vi "Lab Panel V5.24.2.vi"() -> ()   [LabVIEW 2013] (continued)
                            n1486 = TDMS Write(0:w2783, 5:"TEST PASS", 7:w2787, 9:w2786) -> (15:w2789:errorcluster)  [unwired: 2 in, 3 out]
                            n1487 = local write "data file error"(w2789) -> ()
                          }
                          frame #1 {
                            n1488 = Bundle(cluster=w2790, "STATUS"="T-RISE PASS") -> (w2792:T4)  [unwired: 2 in]
                            n1489 = local write "RESULT LAB05-1"(TRUE) -> ()
                            n1490 = local write "DISP LAB05-1"(w2792) -> ()
                          }
                        }
                      }
                      frame False {
                      }
                    }
                  }
                }
              }
              frame #9 {
                # "LAB05-2"
                n1491 = Equal?(x=w2795, y=2) -> (x = y?=w2798:bool)
                n1492 = local read "DISP LAB05-2"() -> (w2800:T4)
                n1493 = Unbundle(w2800) -> ("STATUS"=w2801:string)  [unwired: 2 out]
                n1494 = Equal?(x=w2801, y="RUN") -> (x = y?=w2797:bool)
                n1495 = And(x=w2797, y=w2798) -> (x .and. y?=w2796:bool)
                n1496 = case shown="True" w2796 {
                  tunnel: w2800 -> [_ w2804]
                  tunnel: w2794 -> [_ w2807]
                  frame False {
                  }
                  frame True {
                    n1497 = local read "SET LAB05-2"() -> (w2806:T5)
                    n1498 = local read "TDMS LAB05-2"() -> (w2803:refnum<k34>)
                    n1499 = Unbundle(w2804) -> ("CYCLE"=w2808:dbl)  [unwired: 2 out]
                    n1500 = Unbundle(w2806) -> ("T-RISE mins"=w2805:dbl)  [unwired: 4 out]
                    n1501 = Greater Or Equal?(x=w2808, y=w2807) -> (x >= y?=w2809:bool)
                    n1502 = case shown="True" w2809 {
                      tunnel: w2805 -> [w2812 _]
                      tunnel: w2804 -> [w2811 _]
                      tunnel: w2803 -> [w2810 _]
                      frame True {
                        n1503 = stacked-sequence {
                          tunnel: w2812 -> [w2815 _]
                          tunnel: w2811 -> [_ w2820]
                          tunnel: w2810 -> [w2813 _]
                          frame #0 {
                            n1504 = Build Array("T-RISE") -> (w2817:string[])
                            n1505 = Build Array(w2815) -> (w2816:dbl[])
                            n1506 = TDMS Write(0:w2813, 5:"TEST PASS", 7:w2817, 9:w2816) -> (15:w2819:errorcluster)  [unwired: 2 in, 3 out]
                            n1507 = local write "data file error"(w2819) -> ()
                          }
                          frame #1 {
                            n1508 = Bundle(cluster=w2820, "STATUS"="T-RISE PASS") -> (w2822:T4)  [unwired: 2 in]
                            n1509 = local write "RESULT LAB05-2"(TRUE) -> ()
                            n1510 = local write "DISP LAB05-2"(w2822) -> ()
                          }
                        }
                      }
                      frame False {
                      }
                    }
                  }
                }
              }
            }
          }
          frame #6 {
            # "end test & close test files"
            n1511 = local read "MAIL SETTINGS"() -> (w2828:T7)
            n1512 = Unbundle(w2828) -> ("OUT SERVER ADDRESS"=w2827:string, "FROM ACCOUNT"=w2826:string)  [unwired: 5 out]
            n1513 = stacked-sequence {
              tunnel: w2838 -> [_ _ _ _ _ _ _ _ _ _]
              tunnel: w2839 -> [_ _ _ _ _ _ _ _ _ _]
              tunnel: w2837 -> [_ _ _ _ _ _ _ _ _ _]
              tunnel: w2836 -> [_ _ _ _ _ _ _ _ _ _]
              tunnel: w2835 -> [_ _ _ _ _ _ _ _ _ _]
              tunnel: w2834 -> [_ _ _ _ _ _ _ _ _ _]
              tunnel: w2833 -> [_ _ _ _ _ _ _ _ _ _]
              tunnel: w2832 -> [_ _ _ _ _ _ _ _ _ _]
              tunnel: w2831 -> [_ _ _ _ _ _ _ _ _ _]
              tunnel: w2830 -> [_ _ _ _ _ _ _ _ _ _]
              tunnel: w2827 -> [w2843 w2895 w2943 w2990 w3037 w3084 w3131 w3178 w3225 w3272]
              tunnel: w2826 -> [w2842 w2894 w2942 w2989 w3036 w3083 w3130 w3177 w3224 w3271]
              tunnel: "Mail Test File To:" -> [w2841 w2893 w2941 w2988 w3035 w3082 w3129 w3176 w3223 w3270]
              tunnel: "Mail Test Fail" -> [w2840 w2892 w2940 w2987 w3034 w3081 w3128 w3175 w3222 w3269]
              frame #0 {
                # "LAB01-1"
                n1514 = local read "DISP LAB01-1"() -> (w2847:T4)
                n1515 = local read "run lab01-1"() -> (w2844:bool)
                n1516 = local read "TDMS LAB01-1"() -> (w2845:refnum<k34>)
                n1517 = Unbundle(w2847) -> ("CYCLE"=w2848:dbl, "STATUS"=w2846:string)  [unwired: 1 out]
                n1518 = case shown="True" w2844 {
                  tunnel: w2848 -> [_ w2854]
                  tunnel: w2847 -> [_ w2856]
                  tunnel: w2846 -> [_ w2853]
                  tunnel: w2845 -> [_ w2855]
                  tunnel: w2843 -> [_ w2852]
                  tunnel: w2842 -> [_ w2851]
                  tunnel: w2841 -> [_ w2850]
                  tunnel: w2840 -> [_ w2849]
                  frame False {
                  }
                  frame True {
                    n1519 = Not Equal?(x=w2853, y="RUN") -> (x != y?=w2857:bool)
                    n1520 = Greater?(x=w2854, y=2.0) -> (0:w2859:bool)
                    n1521 = And(x=w2859, y=w2857) -> (x .and. y?=w2858:bool)
                    n1522 = case shown="True" w2858 {
                      tunnel: w2856 -> [_ w2869]
                      tunnel: w2855 -> [_ w2868]
                      tunnel: w2854 -> [_ w2867]
                      tunnel: w2853 -> [_ w2866]
                      tunnel: w2852 -> [_ w2865]
                      tunnel: w2851 -> [_ w2864]
                      tunnel: w2850 -> [_ w2863]
                      tunnel: w2849 -> [_ w2862]
                      frame False {
                      }
                      frame True {
                        n1523 = stacked-sequence {
                          tunnel: w2869 -> [w2873 _ _]
                          tunnel: w2868 -> [_ w2875 _]
                          tunnel: w2867 -> [_ _ _]
                          tunnel: w2866 -> [_ _ w2881]
                          tunnel: w2865 -> [_ _ w2880]
                          tunnel: w2864 -> [_ _ w2879]
                          tunnel: w2863 -> [_ _ w2878]
                          tunnel: w2862 -> [_ _ w2877]
                          frame #0 {
                            w2870 = FALSE
                            n1524 = local write "mail control"("END") -> ()
                            n1525 = Bundle(cluster=w2873) -> (w2872:T4)  [unwired: 3 in]
                            n1526 = local write "DISP LAB01-1"(w2872) -> ()
                            n1527 = local write "O/I  LAB01-1"(w2870) -> ()
                            n1528 = local write "run lab01-1"(w2870) -> ()
                            n1529 = local write "RUN LAB01-1"(w2870) -> ()
                          }
                          frame #1 {
                            n1530 = TDMS Close(11:w2875) -> (0:w2874:errorcluster)  [unwired: 1 in, 1 out]
                            n1531 = local write "data file error"(w2874) -> ()
                          }
                          frame #2 {
                            n1532 = stacked-sequence {
                              tunnel: "LAB01-1" -> [w2883 w2885 _]
                              tunnel: w2881 -> [_ w2891 _]
                              tunnel: w2880 -> [_ w2890 _]
                              tunnel: w2879 -> [_ w2889 _]
                              tunnel: w2878 -> [_ w2888 _]
                              tunnel: w2877 -> [_ w2887 _]
                              frame #0 {
                                n1533 = call "sub vi - defrag tdms v1.vi"("panel id"=w2883) -> ("error out"=w2882:errorcluster)  [unwired: 10 in]
                                n1534 = local write "data file error"(w2882) -> ()
                              }
                              frame #1 {
                                n1535 = Bundle("STATUS"=w2891, "OUT SERVER ADDRESS"=w2890, "FROM ACCOUNT"=w2889, "Mail Test File To:"=w2888, "Mail Test Fail"=w2887) -> (w2884:T26)  [unwired: 1 in]
                                n1536 = call "Save data file (pass-fail) v5.vi"("Input Cluster"=w2884, "panel id"=w2885) -> ("network file save error"=w2886:errorcluster)  [unwired: 8 in, 1 out]
                                n1537 = local write "data file error"(w2886) -> ()
                              }
                              frame #2 {
                              }
                            }
                          }
                        }
                      }
                    }
                  }
                }
              }
              frame #1 {
                # "LAB01-2"
                n1538 = local read "run lab01-2"() -> (w2896:bool)
                n1539 = case shown="True" w2896 {
                  tunnel: w2895 -> [_ w2900]
                  tunnel: w2894 -> [_ w2899]
                  tunnel: w2893 -> [_ w2898]
                  tunnel: w2892 -> [_ w2897]
                  frame False {
                  }
                  frame True {
                    n1540 = local read "DISP LAB01-2"() -> (w2908:T4)
                    n1541 = local read "TDMS LAB01-2"() -> (w2907:refnum<k34>)
                    n1542 = Unbundle(w2908) -> ("CYCLE"=w2902:dbl, "STATUS"=w2901:string)  [unwired: 1 out]
                    n1543 = Not Equal?(x=w2901, y="RUN") -> (x != y?=w2904:bool)
                    n1544 = Greater?(x=w2902, y=2.0) -> (0:w2905:bool)
                    n1545 = And(x=w2905, y=w2904) -> (x .and. y?=w2903:bool)
                    n1546 = case shown="True" w2903 {
                      tunnel: w2908 -> [_ w2917]
                      tunnel: w2907 -> [_ w2916]
                      tunnel: w2902 -> [_ w2915]
                      tunnel: w2901 -> [_ w2914]
                      tunnel: w2900 -> [_ w2913]
                      tunnel: w2899 -> [_ w2912]
                      tunnel: w2898 -> [_ w2911]
                      tunnel: w2897 -> [_ w2910]
                      frame False {
                      }
                      frame True {
                        n1547 = stacked-sequence {
                          tunnel: w2917 -> [w2920 _ _]
                          tunnel: w2916 -> [_ w2922 _]
                          tunnel: w2915 -> [_ _ _]
                          tunnel: w2914 -> [_ _ w2928]
                          tunnel: w2913 -> [_ _ w2927]
                          tunnel: w2912 -> [_ _ w2926]
                          tunnel: w2911 -> [_ _ w2925]
                          tunnel: w2910 -> [_ _ w2924]
                          frame #0 {
                            w2918 = FALSE
                            n1548 = local write "mail control"("END") -> ()
                            n1549 = Bundle(cluster=w2920) -> (w2921:T4)  [unwired: 3 in]
                            n1550 = local write "RUN LAB01-2"(w2918) -> ()
                            n1551 = local write "run lab01-2"(w2918) -> ()
                            n1552 = local write "O/I  LAB01-2"(w2918) -> ()
                            n1553 = local write "DISP LAB01-2"(w2921) -> ()
                          }
                          frame #1 {
                            n1554 = TDMS Close(11:w2922) -> (0:w2923:errorcluster)  [unwired: 1 in, 1 out]
                            n1555 = local write "data file error"(w2923) -> ()
                          }
                          frame #2 {
                            n1556 = stacked-sequence {
                              tunnel: "LAB01-2" -> [w2931 w2932]
                              tunnel: w2928 -> [_ w2937]
                              tunnel: w2927 -> [_ w2936]
                              tunnel: w2926 -> [_ w2935]
                              tunnel: w2925 -> [_ w2934]
                              tunnel: w2924 -> [_ w2933]
                              frame #0 {
                                n1557 = call "sub vi - defrag tdms v1.vi"("panel id"=w2931) -> ("error out"=w2930:errorcluster)  [unwired: 10 in]
                                n1558 = local write "data file error"(w2930) -> ()
                              }
                              frame #1 {
                                n1559 = Bundle("STATUS"=w2937, "OUT SERVER ADDRESS"=w2936, "FROM ACCOUNT"=w2935, "Mail Test File To:"=w2934, "Mail Test Fail"=w2933) -> (w2939:T26)  [unwired: 1 in]
                                n1560 = call "Save data file (pass-fail) v5.vi"("Input Cluster"=w2939, "panel id"=w2932) -> ("network file save error"=w2938:errorcluster)  [unwired: 8 in, 1 out]
                                n1561 = local write "data file error"(w2938) -> ()
                              }
                            }
                          }
                        }
                      }
                    }
                  }
                }
              }
              frame #2 {
                # "LAB02-1"
                n1562 = local read "run lab02-1"() -> (w2944:bool)
                n1563 = case shown="True" w2944 {
                  tunnel: w2943 -> [_ w2948]
                  tunnel: w2942 -> [_ w2947]
                  tunnel: w2941 -> [_ w2946]
                  tunnel: w2940 -> [_ w2945]
                  frame False {
                  }
                  frame True {
                    n1564 = local read "DISP LAB02-1"() -> (w2956:T4)
                    n1565 = Unbundle(w2956) -> ("CYCLE"=w2952:dbl, "STATUS"=w2949:string)  [unwired: 1 out]
                    n1566 = local read "TDMS LAB02-1"() -> (w2955:refnum<k34>)
                    n1567 = Not Equal?(x=w2949, y="RUN") -> (x != y?=w2951:bool)
                    n1568 = Greater?(x=w2952, y=2.0) -> (0:w2953:bool)
                    n1569 = And(x=w2953, y=w2951) -> (x .and. y?=w2950:bool)
                    n1570 = case shown="True" w2950 {
                      tunnel: w2956 -> [_ w2964]
                      tunnel: w2955 -> [_ w2963]
                      tunnel: w2949 -> [_ w2962]
                      tunnel: w2948 -> [_ w2961]
                      tunnel: w2947 -> [_ w2960]
                      tunnel: w2946 -> [_ w2959]
                      tunnel: w2945 -> [_ w2958]
                      frame False {
                      }
                      frame True {
                        n1571 = stacked-sequence {
                          tunnel: w2964 -> [w2967 _ _]
                          tunnel: w2963 -> [_ w2969 _]
                          tunnel: w2962 -> [_ _ w2975]
                          tunnel: w2961 -> [_ _ w2974]
                          tunnel: w2960 -> [_ _ w2973]
                          tunnel: w2959 -> [_ _ w2972]
                          tunnel: w2958 -> [_ _ w2971]
                          frame #0 {
                            w2965 = FALSE
                            n1572 = local write "mail control"("END") -> ()
                            n1573 = Bundle(cluster=w2967) -> (w2968:T4)  [unwired: 3 in]
                            n1574 = local write "O/I  LAB02-1"(w2965) -> ()
                            n1575 = local write "RUN LAB02-1"(w2965) -> ()
                            n1576 = local write "run lab02-1"(w2965) -> ()
                            n1577 = local write "DISP LAB02-1"(w2968) -> ()
                          }
                          frame #1 {
                            n1578 = TDMS Close(11:w2969) -> (0:w2970:errorcluster)  [unwired: 1 in, 1 out]
                            n1579 = local write "data file error"(w2970) -> ()
                          }
                          frame #2 {
                            n1580 = stacked-sequence {
                              tunnel: "LAB02-1" -> [w2978 w2985]
                              tunnel: w2975 -> [_ w2983]
                              tunnel: w2974 -> [_ w2982]
                              tunnel: w2973 -> [_ w2981]
                              tunnel: w2972 -> [_ w2980]
                              tunnel: w2971 -> [_ w2979]
                              frame #0 {
                                n1581 = call "sub vi - defrag tdms v1.vi"("panel id"=w2978) -> ("error out"=w2977:errorcluster)  [unwired: 10 in]
                                n1582 = local write "data file error"(w2977) -> ()
                              }
                              frame #1 {
                                n1583 = Bundle("STATUS"=w2983, "OUT SERVER ADDRESS"=w2982, "FROM ACCOUNT"=w2981, "Mail Test File To:"=w2980, "Mail Test Fail"=w2979) -> (w2984:T26)  [unwired: 1 in]
                                n1584 = call "Save data file (pass-fail) v5.vi"("Input Cluster"=w2984, "panel id"=w2985) -> ("network file save error"=w2986:errorcluster)  [unwired: 8 in, 1 out]
                                n1585 = local write "data file error"(w2986) -> ()
                              }
                            }
                          }
                        }
                      }
                    }
                  }
                }
              }
              frame #3 {
                # "LAB02-2"
                n1586 = local read "run lab02-2"() -> (w2991:bool)
                n1587 = case shown="True" w2991 {
                  tunnel: w2990 -> [_ w2995]
                  tunnel: w2989 -> [_ w2994]
                  tunnel: w2988 -> [_ w2993]
                  tunnel: w2987 -> [_ w2992]
                  frame False {
                  }
                  frame True {
                    n1588 = local read "DISP LAB02-2"() -> (w3003:T4)
                    n1589 = local read "TDMS LAB02-2"() -> (w3002:refnum<k34>)
                    n1590 = Unbundle(w3003) -> ("CYCLE"=w2999:dbl, "STATUS"=w2996:string)  [unwired: 1 out]
                    n1591 = Not Equal?(x=w2996, y="RUN") -> (x != y?=w2998:bool)
                    n1592 = Greater?(x=w2999, y=2.0) -> (0:w3000:bool)
                    n1593 = And(x=w3000, y=w2998) -> (x .and. y?=w2997:bool)
                    n1594 = case shown="True" w2997 {
                      tunnel: w3003 -> [_ w3011]
                      tunnel: w3002 -> [_ w3010]
                      tunnel: w2996 -> [_ w3009]
                      tunnel: w2995 -> [_ w3008]
                      tunnel: w2994 -> [_ w3007]
                      tunnel: w2993 -> [_ w3006]
                      tunnel: w2992 -> [_ w3005]
                      frame False {
                      }
                      frame True {
                        n1595 = stacked-sequence {
                          tunnel: w3011 -> [w3014 _ _]
                          tunnel: w3010 -> [_ w3016 _]
                          tunnel: w3009 -> [_ _ w3022]
                          tunnel: w3008 -> [_ _ w3021]
                          tunnel: w3007 -> [_ _ w3020]
                          tunnel: w3006 -> [_ _ w3019]
                          tunnel: w3005 -> [_ _ w3018]
                          frame #0 {
                            w3012 = FALSE
                            n1596 = local write "mail control"("END") -> ()
                            n1597 = Bundle(cluster=w3014) -> (w3015:T4)  [unwired: 3 in]
                            n1598 = local write "O/I  LAB02-2"(w3012) -> ()
                            n1599 = local write "run lab02-2"(w3012) -> ()
                            n1600 = local write "RUN LAB02-2"(w3012) -> ()
                            n1601 = local write "DISP LAB02-2"(w3015) -> ()
                          }
                          frame #1 {
                            n1602 = TDMS Close(11:w3016) -> (0:w3017:errorcluster)  [unwired: 1 in, 1 out]
                            n1603 = local write "data file error"(w3017) -> ()
                          }
                          frame #2 {
                            n1604 = stacked-sequence {
                              tunnel: "LAB02-2" -> [w3025 w3031]
                              tunnel: w3022 -> [_ w3030]
                              tunnel: w3021 -> [_ w3029]
                              tunnel: w3020 -> [_ w3028]
                              tunnel: w3019 -> [_ w3027]
                              tunnel: w3018 -> [_ w3026]
                              frame #0 {
                                n1605 = call "sub vi - defrag tdms v1.vi"("panel id"=w3025) -> ("error out"=w3024:errorcluster)  [unwired: 10 in]
                                n1606 = local write "data file error"(w3024) -> ()
                              }
                              frame #1 {
                                n1607 = Bundle("STATUS"=w3030, "OUT SERVER ADDRESS"=w3029, "FROM ACCOUNT"=w3028, "Mail Test File To:"=w3027, "Mail Test Fail"=w3026) -> (w3033:T26)  [unwired: 1 in]
                                n1608 = call "Save data file (pass-fail) v5.vi"("Input Cluster"=w3033, "panel id"=w3031) -> ("network file save error"=w3032:errorcluster)  [unwired: 8 in, 1 out]
                                n1609 = local write "data file error"(w3032) -> ()
                              }
                            }
                          }
                        }
                      }
                    }
                  }
                }
              }
              frame #4 {
                # "LAB03-1"
                n1610 = local read "run lab03-1"() -> (w3038:bool)
                n1611 = case shown="True" w3038 {
                  tunnel: w3037 -> [_ w3042]
                  tunnel: w3036 -> [_ w3041]
                  tunnel: w3035 -> [_ w3040]
                  tunnel: w3034 -> [_ w3039]
                  frame False {
                  }
                  frame True {
                    n1612 = local read "DISP LAB03-1"() -> (w3050:T4)
                    n1613 = local read "TDMS LAB03-1"() -> (w3049:refnum<k34>)
                    n1614 = Unbundle(w3050) -> ("CYCLE"=w3046:dbl, "STATUS"=w3043:string)  [unwired: 1 out]
                    n1615 = Not Equal?(x=w3043, y="RUN") -> (x != y?=w3045:bool)
                    n1616 = Greater?(x=w3046, y=2.0) -> (0:w3047:bool)
                    n1617 = And(x=w3047, y=w3045) -> (x .and. y?=w3044:bool)
                    n1618 = case shown="True" w3044 {
                      tunnel: w3050 -> [_ w3058]
                      tunnel: w3049 -> [_ w3057]
                      tunnel: w3043 -> [_ w3056]
                      tunnel: w3042 -> [_ w3055]
                      tunnel: w3041 -> [_ w3054]
                      tunnel: w3040 -> [_ w3053]
                      tunnel: w3039 -> [_ w3052]
                      frame False {
                      }
                      frame True {
                        n1619 = stacked-sequence {
                          tunnel: w3058 -> [w3061 _ _]
                          tunnel: w3057 -> [_ w3063 _]
                          tunnel: w3056 -> [_ _ w3069]
                          tunnel: w3055 -> [_ _ w3068]
                          tunnel: w3054 -> [_ _ w3067]
                          tunnel: w3053 -> [_ _ w3066]
                          tunnel: w3052 -> [_ _ w3065]
                          frame #0 {
                            w3059 = FALSE
                            n1620 = local write "mail control"("END") -> ()
                            n1621 = Bundle(cluster=w3061) -> (w3062:T4)  [unwired: 3 in]
                            n1622 = local write "O/I  LAB03-1"(w3059) -> ()
                            n1623 = local write "run lab03-1"(w3059) -> ()
                            n1624 = local write "RUN LAB03-1"(w3059) -> ()
                            n1625 = local write "DISP LAB03-1"(w3062) -> ()
                          }
                          frame #1 {
                            n1626 = TDMS Close(11:w3063) -> (0:w3064:errorcluster)  [unwired: 1 in, 1 out]
                            n1627 = local write "data file error"(w3064) -> ()
                          }
                          frame #2 {
                            n1628 = stacked-sequence {
                              tunnel: "LAB03-1" -> [w3072 w3078]
                              tunnel: w3069 -> [_ w3077]
                              tunnel: w3068 -> [_ w3076]
                              tunnel: w3067 -> [_ w3075]
                              tunnel: w3066 -> [_ w3074]
                              tunnel: w3065 -> [_ w3073]
                              frame #0 {
                                n1629 = call "sub vi - defrag tdms v1.vi"("panel id"=w3072) -> ("error out"=w3071:errorcluster)  [unwired: 10 in]
                                n1630 = local write "data file error"(w3071) -> ()
                              }
                              frame #1 {
                                n1631 = Bundle("STATUS"=w3077, "OUT SERVER ADDRESS"=w3076, "FROM ACCOUNT"=w3075, "Mail Test File To:"=w3074, "Mail Test Fail"=w3073) -> (w3080:T26)  [unwired: 1 in]
                                n1632 = call "Save data file (pass-fail) v5.vi"("Input Cluster"=w3080, "panel id"=w3078) -> ("network file save error"=w3079:errorcluster)  [unwired: 8 in, 1 out]
                                n1633 = local write "data file error"(w3079) -> ()
                              }
                            }
                          }
                        }
                      }
                    }
                  }
                }
              }
              frame #5 {
                # "LAB03-2"
                n1634 = local read "run lab03-2"() -> (w3085:bool)
                n1635 = case shown="True" w3085 {
                  tunnel: w3084 -> [_ w3089]
                  tunnel: w3083 -> [_ w3088]
                  tunnel: w3082 -> [_ w3087]
                  tunnel: w3081 -> [_ w3086]
                  frame False {
                  }
                  frame True {
                    n1636 = local read "DISP LAB03-2"() -> (w3097:T4)
                    n1637 = Unbundle(w3097) -> ("CYCLE"=w3093:dbl, "STATUS"=w3090:string)  [unwired: 1 out]
                    n1638 = local read "TDMS LAB03-2"() -> (w3096:refnum<k34>)
                    n1639 = Not Equal?(x=w3090, y="RUN") -> (x != y?=w3092:bool)
                    n1640 = Greater?(x=w3093, y=2.0) -> (0:w3094:bool)
                    n1641 = And(x=w3094, y=w3092) -> (x .and. y?=w3091:bool)
                    n1642 = case shown="True" w3091 {
                      tunnel: w3097 -> [_ w3105]
                      tunnel: w3096 -> [_ w3104]
                      tunnel: w3090 -> [_ w3103]
                      tunnel: w3089 -> [_ w3102]
                      tunnel: w3088 -> [_ w3101]
                      tunnel: w3087 -> [_ w3100]
                      tunnel: w3086 -> [_ w3099]
                      frame False {
                      }
                      frame True {
                        n1643 = stacked-sequence {
                          tunnel: w3105 -> [w3108 _ _]
                          tunnel: w3104 -> [_ w3110 _]
                          tunnel: w3103 -> [_ _ w3116]
                          tunnel: w3102 -> [_ _ w3115]
                          tunnel: w3101 -> [_ _ w3114]
                          tunnel: w3100 -> [_ _ w3113]
                          tunnel: w3099 -> [_ _ w3112]
                          frame #0 {
                            w3106 = FALSE
                            n1644 = local write "mail control"("END") -> ()
                            n1645 = Bundle(cluster=w3108) -> (w3109:T4)  [unwired: 3 in]
                            n1646 = local write "RUN LAB03-2"(w3106) -> ()
                            n1647 = local write "O/I  LAB03-2"(w3106) -> ()
                            n1648 = local write "DISP LAB03-2"(w3109) -> ()
                            n1649 = local write "run lab03-2"(w3106) -> ()
                          }
                          frame #1 {
                            n1650 = TDMS Close(11:w3110) -> (0:w3111:errorcluster)  [unwired: 1 in, 1 out]
                            n1651 = local write "data file error"(w3111) -> ()
                          }
                          frame #2 {
                            n1652 = stacked-sequence {
                              tunnel: "LAB03-2" -> [w3119 w3120]
                              tunnel: w3116 -> [_ w3125]
                              tunnel: w3115 -> [_ w3124]
                              tunnel: w3114 -> [_ w3123]
                              tunnel: w3113 -> [_ w3122]
                              tunnel: w3112 -> [_ w3121]
                              frame #0 {
                                n1653 = call "sub vi - defrag tdms v1.vi"("panel id"=w3119) -> ("error out"=w3118:errorcluster)  [unwired: 10 in]
                                n1654 = local write "data file error"(w3118) -> ()
                              }
                              frame #1 {
                                n1655 = Bundle("STATUS"=w3125, "OUT SERVER ADDRESS"=w3124, "FROM ACCOUNT"=w3123, "Mail Test File To:"=w3122, "Mail Test Fail"=w3121) -> (w3127:T26)  [unwired: 1 in]
                                n1656 = call "Save data file (pass-fail) v5.vi"("Input Cluster"=w3127, "panel id"=w3120) -> ("network file save error"=w3126:errorcluster)  [unwired: 8 in, 1 out]
                                n1657 = local write "data file error"(w3126) -> ()
                              }
                            }
                          }
                        }
                      }
                    }
                  }
                }
              }
              frame #6 {
                # "LAB04-1"
                n1658 = local read "run lab04-1"() -> (w3132:bool)
                n1659 = case shown="True" w3132 {
                  tunnel: w3131 -> [_ w3136]
                  tunnel: w3130 -> [_ w3135]
                  tunnel: w3129 -> [_ w3134]
                  tunnel: w3128 -> [_ w3133]
                  frame False {
                  }
                  frame True {
                    n1660 = local read "DISP LAB04-1"() -> (w3144:T4)
                    n1661 = Unbundle(w3144) -> ("CYCLE"=w3140:dbl, "STATUS"=w3137:string)  [unwired: 1 out]
                    n1662 = local read "TDMS LAB04-1"() -> (w3143:refnum<k34>)
                    n1663 = Not Equal?(x=w3137, y="RUN") -> (x != y?=w3139:bool)
                    n1664 = Greater?(x=w3140, y=2.0) -> (0:w3141:bool)
                    n1665 = And(x=w3141, y=w3139) -> (x .and. y?=w3138:bool)
                    n1666 = case shown="True" w3138 {
                      tunnel: w3144 -> [_ w3152]
                      tunnel: w3143 -> [_ w3151]
                      tunnel: w3137 -> [_ w3150]
                      tunnel: w3136 -> [_ w3149]
                      tunnel: w3135 -> [_ w3148]
                      tunnel: w3134 -> [_ w3147]
                      tunnel: w3133 -> [_ w3146]
                      frame False {
                      }
                      frame True {
                        n1667 = stacked-sequence {
                          tunnel: w3152 -> [w3155 _ _]
                          tunnel: w3151 -> [_ w3157 _]
                          tunnel: w3150 -> [_ _ w3163]
                          tunnel: w3149 -> [_ _ w3162]
                          tunnel: w3148 -> [_ _ w3161]
                          tunnel: w3147 -> [_ _ w3160]
                          tunnel: w3146 -> [_ _ w3159]
                          frame #0 {
                            w3153 = FALSE
                            n1668 = local write "mail control"("END") -> ()
                            n1669 = Bundle(cluster=w3155) -> (w3156:T4)  [unwired: 3 in]
                            n1670 = local write "RUN LAB04-1"(w3153) -> ()
                            n1671 = local write "O/I  LAB04-1"(w3153) -> ()
                            n1672 = local write "run lab04-1"(w3153) -> ()
                            n1673 = local write "DISP LAB04-1"(w3156) -> ()
                          }
                          frame #1 {
                            n1674 = TDMS Close(11:w3157) -> (0:w3158:errorcluster)  [unwired: 1 in, 1 out]
                            n1675 = local write "data file error"(w3158) -> ()
                          }
                          frame #2 {
                            n1676 = stacked-sequence {
                              tunnel: "LAB04-1" -> [w3166 w3167]
                              tunnel: w3163 -> [_ w3172]
                              tunnel: w3162 -> [_ w3171]
                              tunnel: w3161 -> [_ w3170]
                              tunnel: w3160 -> [_ w3169]
                              tunnel: w3159 -> [_ w3168]
                              frame #0 {
                                n1677 = call "sub vi - defrag tdms v1.vi"("panel id"=w3166) -> ("error out"=w3165:errorcluster)  [unwired: 10 in]
                                n1678 = local write "data file error"(w3165) -> ()
                              }
                              frame #1 {
                                n1679 = Bundle("STATUS"=w3172, "OUT SERVER ADDRESS"=w3171, "FROM ACCOUNT"=w3170, "Mail Test File To:"=w3169, "Mail Test Fail"=w3168) -> (w3174:T26)  [unwired: 1 in]
                                n1680 = call "Save data file (pass-fail) v5.vi"("Input Cluster"=w3174, "panel id"=w3167) -> ("network file save error"=w3173:errorcluster)  [unwired: 8 in, 1 out]
                                n1681 = local write "data file error"(w3173) -> ()
                              }
                            }
                          }
                        }
                      }
                    }
                  }
                }
              }
              frame #7 {
                # "LAB04-2"
                n1682 = local read "run lab04-2"() -> (w3179:bool)
                n1683 = case shown="True" w3179 {
                  tunnel: w3178 -> [_ w3183]
                  tunnel: w3177 -> [_ w3182]
                  tunnel: w3176 -> [_ w3181]
                  tunnel: w3175 -> [_ w3180]
                  frame False {
                  }
                  frame True {
                    n1684 = local read "DISP LAB04-2"() -> (w3191:T4)
                    n1685 = Unbundle(w3191) -> ("CYCLE"=w3187:dbl, "STATUS"=w3184:string)  [unwired: 1 out]
                    n1686 = Not Equal?(x=w3184, y="RUN") -> (x != y?=w3186:bool)
                    n1687 = local read "TDMS LAB04-2"() -> (w3190:refnum<k34>)
                    n1688 = Greater?(x=w3187, y=2.0) -> (0:w3188:bool)
                    n1689 = And(x=w3188, y=w3186) -> (x .and. y?=w3185:bool)
                    n1690 = case shown="True" w3185 {
                      tunnel: w3191 -> [_ w3199]
                      tunnel: w3190 -> [_ w3198]
                      tunnel: w3184 -> [_ w3197]
                      tunnel: w3183 -> [_ w3196]
                      tunnel: w3182 -> [_ w3195]
                      tunnel: w3181 -> [_ w3194]
                      tunnel: w3180 -> [_ w3193]
                      frame False {
                      }
                      frame True {
                        n1691 = stacked-sequence {
                          tunnel: w3199 -> [w3202 _ _]
                          tunnel: w3198 -> [_ w3204 _]
                          tunnel: w3197 -> [_ _ w3210]
                          tunnel: w3196 -> [_ _ w3209]
                          tunnel: w3195 -> [_ _ w3208]
                          tunnel: w3194 -> [_ _ w3207]
                          tunnel: w3193 -> [_ _ w3206]
                          frame #0 {
                            w3200 = FALSE
                            n1692 = local write "mail control"("END") -> ()
                            n1693 = Bundle(cluster=w3202) -> (w3203:T4)  [unwired: 3 in]
                            n1694 = local write "O/I  LAB04-2"(w3200) -> ()
                            n1695 = local write "RUN LAB04-2"(w3200) -> ()
                            n1696 = local write "run lab04-2"(w3200) -> ()
                            n1697 = local write "DISP LAB04-2"(w3203) -> ()
                          }
                          frame #1 {
                            n1698 = TDMS Close(11:w3204) -> (0:w3205:errorcluster)  [unwired: 1 in, 1 out]
                            n1699 = local write "data file error"(w3205) -> ()
                          }
                          frame #2 {
                            n1700 = stacked-sequence {
                              tunnel: "LAB04-2" -> [w3213 w3214]
                              tunnel: w3210 -> [_ w3219]
                              tunnel: w3209 -> [_ w3218]
                              tunnel: w3208 -> [_ w3217]
                              tunnel: w3207 -> [_ w3216]
                              tunnel: w3206 -> [_ w3215]
                              frame #0 {
                                n1701 = call "sub vi - defrag tdms v1.vi"("panel id"=w3213) -> ("error out"=w3212:errorcluster)  [unwired: 10 in]
                                n1702 = local write "data file error"(w3212) -> ()
                              }
                              frame #1 {
                                n1703 = Bundle("STATUS"=w3219, "OUT SERVER ADDRESS"=w3218, "FROM ACCOUNT"=w3217, "Mail Test File To:"=w3216, "Mail Test Fail"=w3215) -> (w3221:T26)  [unwired: 1 in]
                                n1704 = call "Save data file (pass-fail) v5.vi"("Input Cluster"=w3221, "panel id"=w3214) -> ("network file save error"=w3220:errorcluster)  [unwired: 8 in, 1 out]
                                n1705 = local write "data file error"(w3220) -> ()
                              }
                            }
                          }
                        }
                      }
                    }
                  }
                }
              }
              frame #8 {
                # "LAB05-1"
                n1706 = local read "run lab05-1"() -> (w3226:bool)
                n1707 = case shown="True" w3226 {
                  tunnel: w3225 -> [_ w3230]
                  tunnel: w3224 -> [_ w3229]
                  tunnel: w3223 -> [_ w3228]
                  tunnel: w3222 -> [_ w3227]
                  frame False {
                  }
                  frame True {
                    n1708 = local read "DISP LAB05-1"() -> (w3238:T4)
                    n1709 = Unbundle(w3238) -> ("CYCLE"=w3234:dbl, "STATUS"=w3231:string)  [unwired: 1 out]
                    n1710 = Not Equal?(x=w3231, y="RUN") -> (x != y?=w3233:bool)
                    n1711 = local read "TDMS LAB05-1"() -> (w3237:refnum<k34>)
                    n1712 = Greater?(x=w3234, y=2.0) -> (0:w3235:bool)
                    n1713 = And(x=w3235, y=w3233) -> (x .and. y?=w3232:bool)
                    n1714 = case shown="True" w3232 {
                      tunnel: w3238 -> [_ w3246]
                      tunnel: w3237 -> [_ w3245]
                      tunnel: w3231 -> [_ w3244]
                      tunnel: w3230 -> [_ w3243]
                      tunnel: w3229 -> [_ w3242]
                      tunnel: w3228 -> [_ w3241]
                      tunnel: w3227 -> [_ w3240]
                      frame False {
                      }
                      frame True {
                        n1715 = stacked-sequence {
                          tunnel: w3246 -> [w3249 _ _]
                          tunnel: w3245 -> [_ w3251 _]
                          tunnel: w3244 -> [_ _ w3257]
                          tunnel: w3243 -> [_ _ w3256]
                          tunnel: w3242 -> [_ _ w3255]
                          tunnel: w3241 -> [_ _ w3254]
                          tunnel: w3240 -> [_ _ w3253]
                          frame #0 {
                            w3247 = FALSE
                            n1716 = local write "mail control"("END") -> ()
                            n1717 = Bundle(cluster=w3249) -> (w3250:T4)  [unwired: 3 in]
                            n1718 = local write "O/I  LAB05-1"(w3247) -> ()
                            n1719 = local write "RUN LAB05-1"(w3247) -> ()
                            n1720 = local write "run lab05-1"(w3247) -> ()
                            n1721 = local write "DISP LAB05-1"(w3250) -> ()
                          }
                          frame #1 {
                            n1722 = TDMS Close(11:w3251) -> (0:w3252:errorcluster)  [unwired: 1 in, 1 out]
                            n1723 = local write "data file error"(w3252) -> ()
                          }
                          frame #2 {
                            n1724 = stacked-sequence {
                              tunnel: "LAB05-1" -> [w3260 w3266]
                              tunnel: w3257 -> [_ w3265]
                              tunnel: w3256 -> [_ w3264]
                              tunnel: w3255 -> [_ w3263]
                              tunnel: w3254 -> [_ w3262]
                              tunnel: w3253 -> [_ w3261]
                              frame #0 {
                                n1725 = call "sub vi - defrag tdms v1.vi"("panel id"=w3260) -> ("error out"=w3259:errorcluster)  [unwired: 10 in]
                                n1726 = local write "data file error"(w3259) -> ()
                              }
                              frame #1 {
                                n1727 = Bundle("STATUS"=w3265, "OUT SERVER ADDRESS"=w3264, "FROM ACCOUNT"=w3263, "Mail Test File To:"=w3262, "Mail Test Fail"=w3261) -> (w3268:T26)  [unwired: 1 in]
                                n1728 = call "Save data file (pass-fail) v5.vi"("Input Cluster"=w3268, "panel id"=w3266) -> ("network file save error"=w3267:errorcluster)  [unwired: 8 in, 1 out]
                                n1729 = local write "data file error"(w3267) -> ()
                              }
                            }
                          }
                        }
                      }
                    }
                  }
                }
              }
              frame #9 {
                # "LAB05-2"
                n1730 = local read "run lab05-2"() -> (w3273:bool)
                n1731 = case shown="True" w3273 {
                  tunnel: w3272 -> [_ w3277]
                  tunnel: w3271 -> [_ w3276]
                  tunnel: w3270 -> [_ w3275]
                  tunnel: w3269 -> [_ w3274]
                  frame False {
                  }
                  frame True {
                    n1732 = local read "DISP LAB05-2"() -> (w3285:T4)
                    n1733 = Unbundle(w3285) -> ("CYCLE"=w3281:dbl, "STATUS"=w3278:string)  [unwired: 1 out]
                    n1734 = Not Equal?(x=w3278, y="RUN") -> (x != y?=w3280:bool)
                    n1735 = local read "TDMS LAB05-2"() -> (w3284:refnum<k34>)
                    n1736 = Greater?(x=w3281, y=2.0) -> (0:w3282:bool)
                    n1737 = And(x=w3282, y=w3280) -> (x .and. y?=w3279:bool)
                    n1738 = case shown="True" w3279 {
                      tunnel: w3285 -> [_ w3293]
                      tunnel: w3284 -> [_ w3292]
                      tunnel: w3278 -> [_ w3291]
                      tunnel: w3277 -> [_ w3290]
                      tunnel: w3276 -> [_ w3289]
                      tunnel: w3275 -> [_ w3288]
                      tunnel: w3274 -> [_ w3287]
                      frame False {
                      }
                      frame True {
                        n1739 = stacked-sequence {
                          tunnel: w3293 -> [w3296 _ _]
                          tunnel: w3292 -> [_ w3298 _]
                          tunnel: w3291 -> [_ _ w3304]
                          tunnel: w3290 -> [_ _ w3303]
                          tunnel: w3289 -> [_ _ w3302]
                          tunnel: w3288 -> [_ _ w3301]
                          tunnel: w3287 -> [_ _ w3300]
                          frame #0 {
                            w3294 = FALSE
                            n1740 = local write "mail control"("END") -> ()
                            n1741 = Bundle(cluster=w3296) -> (w3297:T4)  [unwired: 3 in]
                            n1742 = local write "RUN LAB05-2"(w3294) -> ()
                            n1743 = local write "O/I  LAB05-2"(w3294) -> ()
                            n1744 = local write "run lab05-2"(w3294) -> ()
                            n1745 = local write "DISP LAB05-2"(w3297) -> ()
                          }
                          frame #1 {
                            n1746 = TDMS Close(11:w3298) -> (0:w3299:errorcluster)  [unwired: 1 in, 1 out]
                            n1747 = local write "data file error"(w3299) -> ()
                          }
                          frame #2 {
                            n1748 = stacked-sequence {
                              tunnel: "LAB05-2" -> [w3307 w3313]
                              tunnel: w3304 -> [_ w3312]
                              tunnel: w3303 -> [_ w3311]
                              tunnel: w3302 -> [_ w3310]
                              tunnel: w3301 -> [_ w3309]
                              tunnel: w3300 -> [_ w3308]
                              frame #0 {
                                n1749 = call "sub vi - defrag tdms v1.vi"("panel id"=w3307) -> ("error out"=w3306:errorcluster)  [unwired: 10 in]
                                n1750 = local write "data file error"(w3306) -> ()
                              }
                              frame #1 {
                                n1751 = Bundle("STATUS"=w3312, "OUT SERVER ADDRESS"=w3311, "FROM ACCOUNT"=w3310, "Mail Test File To:"=w3309, "Mail Test Fail"=w3308) -> (w3315:T26)  [unwired: 1 in]
                                n1752 = call "Save data file (pass-fail) v5.vi"("Input Cluster"=w3315, "panel id"=w3313) -> ("network file save error"=w3314:errorcluster)  [unwired: 8 in, 1 out]
                                n1753 = local write "data file error"(w3314) -> ()
                              }
                            }
                          }
                        }
                      }
                    }
                  }
                }
              }
            }
            n1754 = local read "Network Directory"() -> (w2829:path)
            n1755 = global write "Global 1.vi" "Network Drive"(w2829) -> ()
          }
          frame #7 {
            # "disable functions"
            n1756 = stacked-sequence {
              tunnel: w3325 -> [w3339 _ w3396]
              tunnel: w3324 -> [w3334 _ w3395]
              tunnel: w3323 -> [w3333 _ w3394]
              tunnel: w3322 -> [w3331 _ w3393]
              tunnel: w3321 -> [w3332 _ w3392]
              tunnel: w3320 -> [_ w3356 w3391]
              tunnel: w3319 -> [_ w3357 w3390]
              tunnel: w3318 -> [_ w3358 w3389]
              tunnel: w3317 -> [_ w3359 w3388]
              tunnel: w3316 -> [_ w3360 w3387]
              frame #0 {
                n1757 = Select(t=2, s=w3331, f=0) -> (s? t:f=w3327:i32)
                n1758 = Select(t=2, s=w3333, f=0) -> (s? t:f=w3328:i32)
                n1759 = Select(t=2, s=w3332, f=0) -> (s? t:f=w3326:i32)
                n1760 = Select(t=2, s=w3339, f=0) -> (s? t:f=w3330:i32)
                n1761 = Select(t=2, s=w3334, f=0) -> (s? t:f=w3329:i32)
                n1762 = property on="SELECT LAB02-2" class="RadioBtnsControl (strict)"("DisabledEnum"=w3327) -> ()  [unwired: 2 in, 2 out]
                n1763 = property on="SELECT LAB02-1" class="RadioBtnsControl (strict)"("DisabledEnum"=w3328) -> ()  [unwired: 2 in, 2 out]
                n1764 = property on="SELECT LAB03-1" class="RadioBtnsControl (strict)"("DisabledEnum"=w3326) -> ()  [unwired: 2 in, 2 out]
                n1765 = property on="SELECT LAB01-1" class="RadioBtnsControl (strict)"("DisabledEnum"=w3330) -> ()  [unwired: 2 in, 2 out]
                n1766 = property on="SELECT LAB01-2" class="RadioBtnsControl (strict)"("DisabledEnum"=w3329) -> ()  [unwired: 2 in, 2 out]
                n1767 = Not(x=w3339) -> (.not. x?=w3340:bool)
                n1768 = property on="RESULT LAB01-1" class="Bool (strict)"("Visible"=w3340) -> ()  [unwired: 2 in, 2 out]
                n1769 = Not(x=w3334) -> (.not. x?=w3338:bool)
                n1770 = Not(x=w3333) -> (.not. x?=w3337:bool)
                n1771 = Not(x=w3331) -> (.not. x?=w3336:bool)
                n1772 = property on="RESULT LAB01-2" class="Bool (strict)"("Visible"=w3338) -> ()  [unwired: 2 in, 2 out]
                n1773 = Not(x=w3332) -> (.not. x?=w3335:bool)
                n1774 = property on="RESULT LAB02-1" class="Bool (strict)"("Visible"=w3337) -> ()  [unwired: 2 in, 2 out]
                n1775 = property on="RESULT LAB02-2" class="Bool (strict)"("Visible"=w3336) -> ()  [unwired: 2 in, 2 out]
                n1776 = property on="RESULT LAB03-1" class="Bool (strict)"("Visible"=w3335) -> ()  [unwired: 2 in, 2 out]
                n1777 = property on="SET LAB01-1" class="Clust (strict)"("DisabledEnum"=w3330) -> ()  [unwired: 2 in, 2 out]
                n1778 = property on="SET LAB01-2" class="Clust (strict)"("DisabledEnum"=w3329) -> ()  [unwired: 2 in, 2 out]
                n1779 = property on="SET LAB02-1" class="Clust (strict)"("DisabledEnum"=w3328) -> ()  [unwired: 2 in, 2 out]
                n1780 = property on="SET LAB02-2" class="Clust (strict)"("DisabledEnum"=w3327) -> ()  [unwired: 2 in, 2 out]
                n1781 = property on="SET LAB03-1" class="Clust (strict)"("DisabledEnum"=w3326) -> ()  [unwired: 2 in, 2 out]
                n1782 = property on="O/I  LAB01-1" class="Bool (strict)"("DisabledEnum"=w3330) -> ()  [unwired: 2 in, 2 out]
                n1783 = property on="O/I  LAB01-2" class="Bool (strict)"("DisabledEnum"=w3329) -> ()  [unwired: 2 in, 2 out]
